vi "ExtractBands.vi"(8 "Task":T1(ring)=enum."Grab Bands", 10 "lines":i32, 11 "plot in":cluster{dbl, "dt":dbl, "Y":dbl[]}[](array[cluster])) -> (2 "Starting line":i32, 3 "plot out":cluster{dbl, "dt":dbl, "Y":dbl[]}[](array[cluster]))   [LabVIEW 2022 SP3]
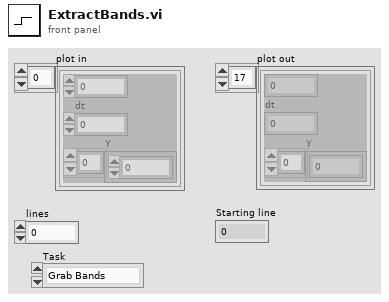
[diagram p1: front panel]
types:
  T1 = enum16{"Grab Lines", "Grab Bands", "Grab Centroids"}
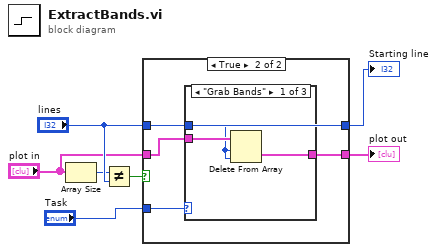
[diagram p0: block diagram]
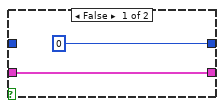
[diagram p2: hidden frame]
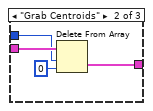
[diagram p3: hidden frame]
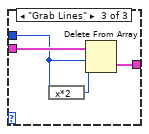
[diagram p4: hidden frame]
diagram:
  n1 = Array Size(array="plot in") -> (size(s)=w2:i32)
  n2 = Not Equal?(x=w2, y="lines") -> (x != y?=w6:bool)
  n3 = case shown="True" w6 {
    tunnel: "plot in" -> [w9 w13]
    tunnel: "lines" -> [_ w11]
    tunnel: [w9 w12] -> w5
    tunnel: [0 w11] -> w7
    tunnel: "Task" -> [_ w10]
    frame False {
    }
    frame True {
      n4 = case shown="\"Grab Bands\"" w10 {
        tunnel: w13 -> [w16 w20 w24]
        tunnel: [w15 w19 w23] -> w12
        tunnel: w11 -> [w14 w18 w22]
        frame "Grab Bands" {
          n5 = Delete From Array(array=w16, length=w14, index=w14) -> (deleted portion=w15:cluster{dbl, "dt":dbl, "Y":dbl[]}[])  [unwired: 1 out]
        }
        frame "Grab Centroids" {
          n6 = Delete From Array(array=w20, length=w18, index=0) -> (deleted portion=w19:cluster{dbl, "dt":dbl, "Y":dbl[]}[])  [unwired: 1 out]
        }
        frame "Grab Lines" {
          n7 = expression code="x*2"(w22) -> (w21:i32)
          n8 = Delete From Array(array=w24, length=w22, index=w21) -> (deleted portion=w23:cluster{dbl, "dt":dbl, "Y":dbl[]}[])  [unwired: 1 out]
        }
      }
    }
  }
  "Starting line" <- w7
  "plot out" <- w5
